vi "(SubVI) Calculate pFC Slope_YCC.vi"(3 "given-power":dbl, 5 "Slope":dbl[](array[numeric])=[0.09, 0.75], 6 "power":dbl[](array[numeric])=[290.0, 1200.0]) -> (1 "Cal-slope (V/um)":dbl)   [LabVIEW 2014]
uses:
  <vilib>/Analysis/NI_AALPro.lvlib
panel:
  out "intercept":dbl
  out "slope":dbl
  out "XY Graph":T1(graph)
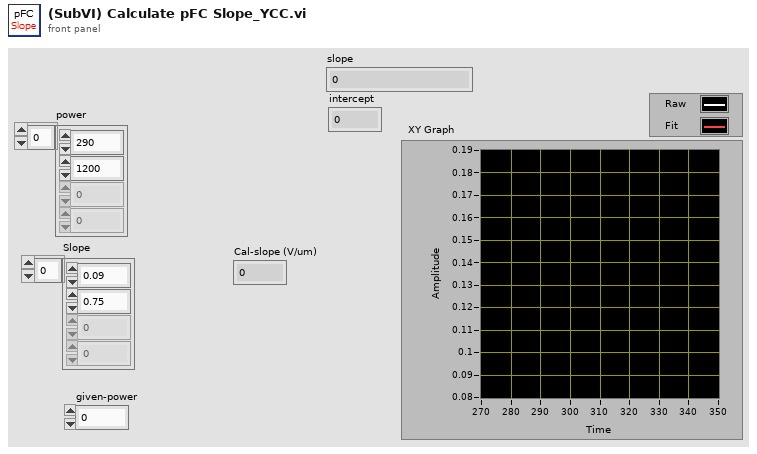
[diagram p1: front panel]
types:
  T1 = cluster{"power":dbl[], "Best Linear Fit":dbl[]}[]
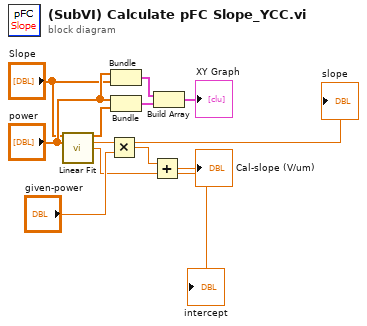
[diagram p0: block diagram]
diagram:
  n1 = call <vilib>:"Linear Fit.vi"("Y"="Slope", "X"="power") -> ("Best Linear Fit"=w10:dbl[], "slope"=w4:dbl, "intercept"=w2:dbl)  [unwired: 9 in, 2 out]
  "slope" <- w4
  "intercept" <- w2
  n2 = Multiply(x=w4, y="given-power") -> (x*y=w3:dbl)
  n3 = Bundle("power"="power", "Slope"="Slope") -> (w8:cluster{"power":dbl[], "Slope":dbl[]})  [unwired: 1 in]
  n4 = Bundle("power"="power", "Best Linear Fit"=w10) -> (w7:cluster{"power":dbl[], "Best Linear Fit":dbl[]})  [unwired: 1 in]
  n5 = Add(x=w3, y=w2) -> (x+y=→"Cal-slope (V/um)":dbl)
  n6 = Build Array(w8, w7) -> (→"XY Graph":T1)
